vi "Set Frequency.vi"(8 "error in (no error)":errorcluster, 10 "Frequency":dbl format="%#_6pHz", 11 "Red Pitaya Lock-in Driver in":refnum<class "Red Pitaya Lock-in Driver.lvclass">) -> (0 "error out":errorcluster, 3 "Red Pitaya Lock-in Driver out":refnum<class "Red Pitaya Lock-in Driver.lvclass">)   [LabVIEW 2015, in "Red Pitaya Lock-in Driver.lvclass"]
uses:
  Red Pitaya Lock-in Driver.lvclass
  Red Pitaya Lock-in Driver.lvclass/Red Pitaya Lock-in Driver.ctl
  Read RP Instrument.vi
  Write RP Instrument.vi
  RP Instrument/RP Instrument.lvclass
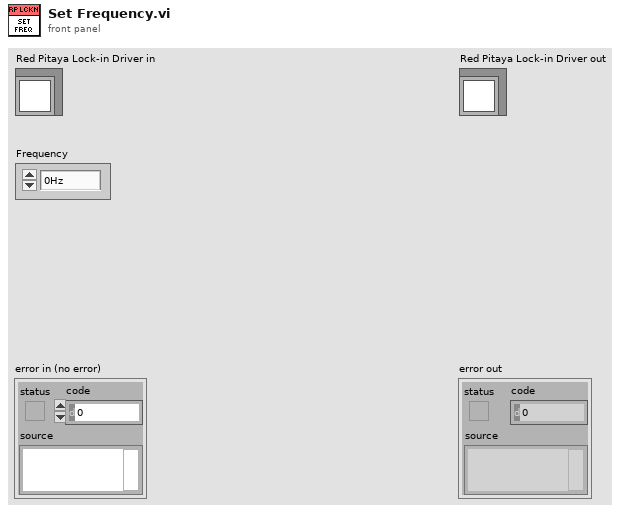
[diagram p1: front panel]
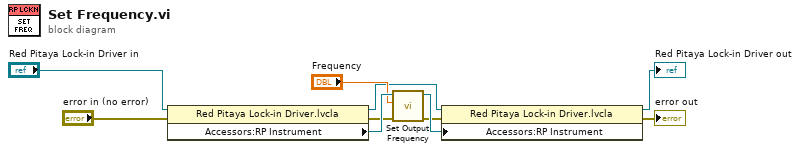
[diagram p0: block diagram]
diagram:
  n1 = property class="Red Pitaya Lock-in Driver.lvcla"(reference="Red Pitaya Lock-in Driver in", error in="error in (no error)") -> (reference out=w6:refnum<class "Red Pitaya Lock-in Driver.lvclass">, error out=w1:errorcluster, "Accessors:RP Instrument"=w8:refnum<class "RP Instrument.lvclass">)
  n2 = call-dynamic "Set Output Frequency.vi"("error in (no error)"=w1, "Frequency"="Frequency", "RP Instrument in"=w8) -> ("error out"=w2:errorcluster, "RP Instrument out"=w5:refnum<class "RP Instrument.lvclass">)  [unwired: 7 in]
  n3 = property class="Red Pitaya Lock-in Driver.lvcla"(reference=w6, error in=w2, "Accessors:RP Instrument"=w5) -> (reference out=→"Red Pitaya Lock-in Driver out":refnum<class "Red Pitaya Lock-in Driver.lvclass">, error out=→"error out":errorcluster)
